vi "Pose_RelativeTo.vi"(9 "other POSE":T1, 11 "in POSE":T1) -> (3 "out POSE":T1)   [LabVIEW 2019, in "PathExecution_Library.lvlib"]
uses:
  PathExecution_Library.lvlib
  POSE.ctl
  TRANSLATION.ctl
  ROTATION.ctl
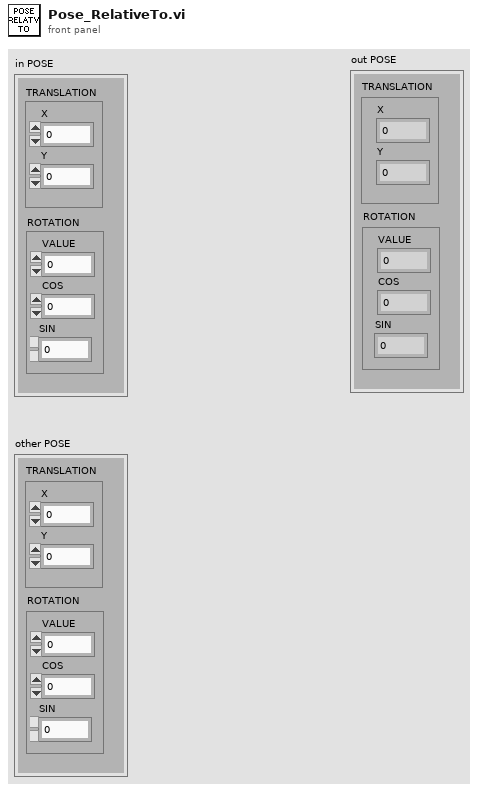
[diagram p1: front panel]
types:
  T1 = typedef "PathExecution_Library.lvlib/POSE.ctl" = cluster{"TRANSLATION":T2, "ROTATION":T3}
  T2 = typedef "PathExecution_Library.lvlib/TRANSLATION.ctl" = cluster{"X":dbl, "Y":dbl}
  T3 = typedef "PathExecution_Library.lvlib/ROTATION.ctl" = cluster{"VALUE":dbl, "COS":dbl, "SIN":dbl}
  T4 = typedef "PathExecution_Library.lvlib/TRANSFORM.ctl" = cluster{"TRANSLATION":T2, "ROTATION":T3}
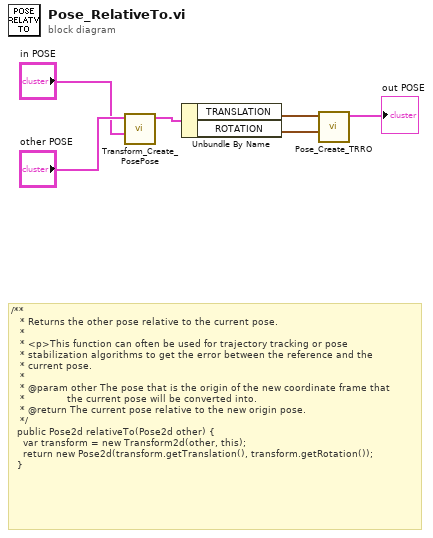
[diagram p0: block diagram]
diagram:
  # "/**\n   * Returns the other pose relative to the current pose.\n   *\n   * <p>This function can often be used for trajectory tracking or pose\n   * stabilization algorithms to get the error between the reference and the\n   * current pose.\n   *\n   * @param other The pose that is the origin of the new coordinate frame that\n   *              the current pose will be converted into.\n   * @return The current pose relative to the new origin pose.\n   */\n  public Pose2d relativeTo(Pose2d other) {\n    var transform = new Transform2d(other, this);\n    return new Pose2d(transform.getTranslation(), transform.getRotation());\n  }"
  n1 = call "Transform_Create_PosePose.vi"("last POSE"="in POSE", "initial POSE"="other POSE") -> ("TRANSFORM"=w6:T4)  [unwired: 9 in]
  n2 = Unbundle By Name(w6) -> ("TRANSLATION"=w2:T2, "ROTATION"=w1:T3)
  n3 = call "Pose_Create_TRRO.vi"("ROTATION"=w1, "TRANSLATION"=w2) -> ("out POSe"=→"out POSE":T1)  [unwired: 9 in]
